vi "SineWaveGraph(WhileLoop).vi"() -> ()   [LabVIEW 2015]
panel:
  out "Array":dbl[](array[numeric])
  out "Waveform Graph":cluster{dbl, dbl, dbl[]}(graph)
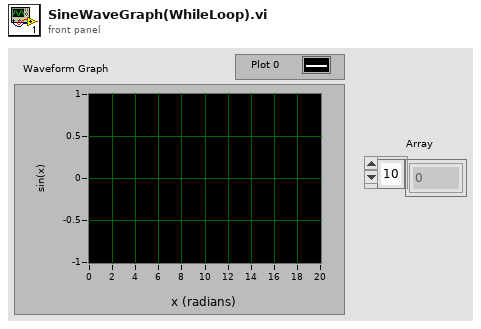
[diagram p1: front panel]
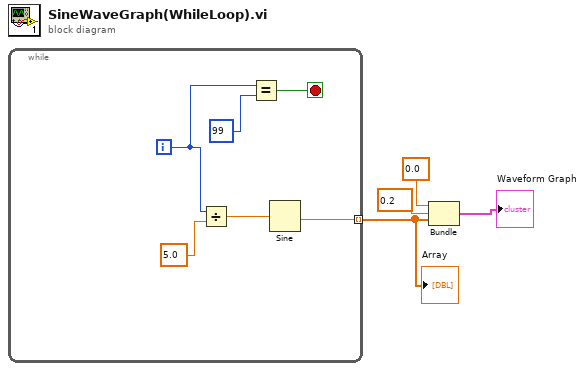
[diagram p0: block diagram]
diagram:
  n1 = while {
    tunnel: [w5] -> w1 mode=indexing
    i -> [w7]
    stop <- w9 stop-if-true
    n2 = Divide(x=w7, y=5.0) -> (x/y=w6:dbl)
    n3 = Equal?(x=w7, y=99) -> (x = y?=w9:bool)
    n4 = Sine(x=w6) -> (sin(x)=w5:dbl)
  }
  "Array" <- w1
  n5 = Bundle(0.0, 0.2, w1) -> (→"Waveform Graph":cluster{dbl, dbl, dbl[]})  [unwired: 1 in]
